vi "Converter.vi"(8 "Error In":errorcluster, 10 "Numeric Control":i32) -> (0 "Error Out":errorcluster, 2 "Digit":T1)   [LabVIEW 2012]
uses:
  Black Display.ctl
  Vertical.ctl
  Horizontal.ctl
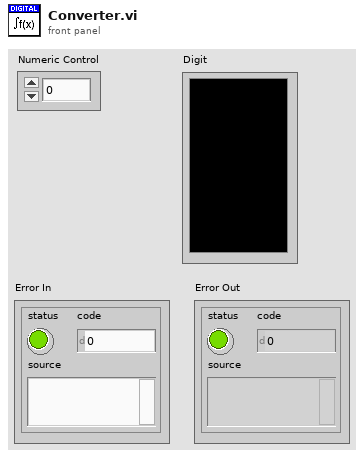
[diagram p1: front panel]
types:
  T1 = typedef "Black Display.ctl" = cluster{"V1":T2, "V2":T2, "H1":T3, "H2":T3, "V3":T2, "V4":T2, "H3":T3}
  T2 = typedef "Vertical.ctl" = bool
  T3 = typedef "Horizontal.ctl" = bool
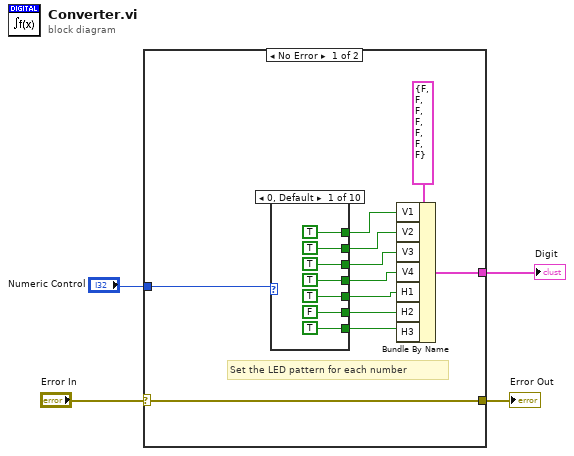
[diagram p0: block diagram]
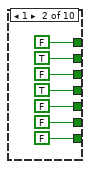
[diagram p2: hidden frame]
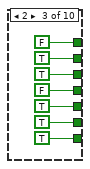
[diagram p3: hidden frame]
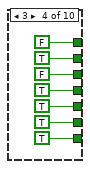
[diagram p4: hidden frame]
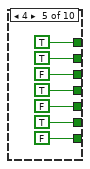
[diagram p5: hidden frame]
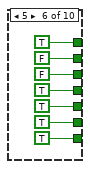
[diagram p6: hidden frame]
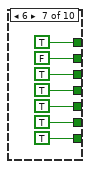
[diagram p7: hidden frame]
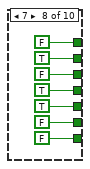
[diagram p8: hidden frame]
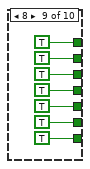
[diagram p9: hidden frame]
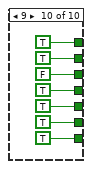
[diagram p10: hidden frame]
diagram:
  n1 = case shown="No Error" "Error In" {
    selector: "Error In" -> [w6 w86]
    tunnel: [w7 _] -> w4
    tunnel: [w6 w86] -> w2
    tunnel: "Numeric Control" -> [w5 _]
    frame No Error {
      # "Set the LED pattern for each number"
      n2 = case shown="0, Default" w5 {
        tunnel: [TRUE FALSE FALSE FALSE TRUE TRUE TRUE FALSE TRUE TRUE] -> w15
        tunnel: [TRUE TRUE TRUE TRUE TRUE FALSE FALSE TRUE TRUE TRUE] -> w14
        tunnel: [TRUE FALSE TRUE FALSE FALSE FALSE TRUE FALSE TRUE FALSE] -> w13
        tunnel: [TRUE TRUE FALSE TRUE TRUE TRUE TRUE TRUE TRUE TRUE] -> w12
        tunnel: [TRUE FALSE TRUE TRUE FALSE TRUE TRUE TRUE TRUE TRUE] -> w11
        tunnel: [FALSE FALSE TRUE TRUE TRUE TRUE TRUE FALSE TRUE TRUE] -> w10
        tunnel: [TRUE FALSE TRUE TRUE FALSE TRUE TRUE FALSE TRUE TRUE] -> w9
        frame 0, Default {
        }
        frame 1 {
        }
        frame 2 {
        }
        frame 3 {
        }
        frame 4 {
        }
        frame 5 {
        }
        frame 6 {
        }
        frame 7 {
        }
        frame 8 {
        }
        frame 9 {
        }
      }
      n3 = Bundle By Name(cluster=T1 {"V1"=FALSE, "V2"=FALSE, "H1"=FALSE, "H2"=FALSE, "V3"=FALSE, "V4"=FALSE, "H3"=FALSE} ("Digit 2"), "V1"=w15, "V2"=w14, "V3"=w13, "V4"=w12, "H1"=w11, "H2"=w10, "H3"=w9) -> (w7:T1)
    }
    frame Error {
    }
  }
  "Error Out" <- w2
  "Digit" <- w4
